vi "Create.vi"(8 "error in (no error)":errorcluster, 11 "Threads":refnum<class "Thread.lvclass">[](array[class])) -> (0 "error out":errorcluster, 3 "Thread Manager out":refnum<class "Thread Manager.lvclass">)   [LabVIEW 2017, in "DSF Core.lvlib" / "Thread Manager.lvclass"]
uses:
  Thread Manager.lvclass
  Thread/Thread.lvclass
  Thread Manager.lvclass/Thread Manager.ctl
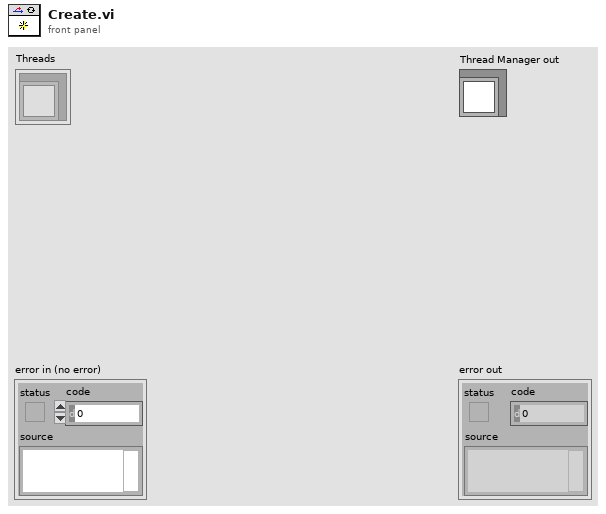
[diagram p1: front panel]
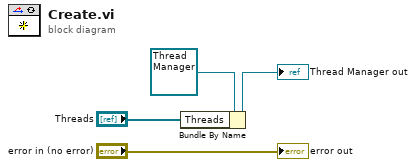
[diagram p0: block diagram]
diagram:
  n1 = Bundle By Name(cluster=refnum<class "Thread Manager.lvclass"> refnum ("Thread Manager in"), "Threads"="Threads") -> (→"Thread Manager out":refnum<class "Thread Manager.lvclass">)
  "error out" <- "error in (no error)"
